vi "Write Boolean Value.vi"(8 "error in (no error)":errorcluster, 10 "Visible?":bool, 11 "Boolean Assertion in":refnum<class "Boolean Assertion.lvclass">) -> (0 "error out":errorcluster, 3 "Boolean Assertion out":refnum<class "Boolean Assertion.lvclass">)   [LabVIEW 2020, in "MacroAssert.lvlib" / "Boolean Assertion.lvclass"]
uses:
  Boolean Assertion.lvclass
  Boolean Assertion.lvclass/Boolean Assertion.ctl
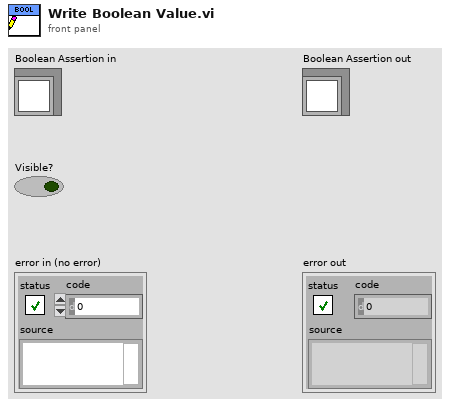
[diagram p1: front panel]
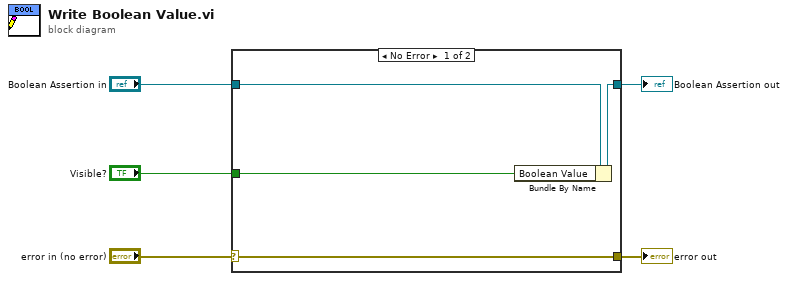
[diagram p0: block diagram]
diagram:
  n1 = case shown="No Error" "error in (no error)" {
    selector: "error in (no error)" -> [w9 w10]
    tunnel: [w9 w10] -> w4
    tunnel: [w7 w11] -> w2
    tunnel: "Boolean Assertion in" -> [w8 w11]
    tunnel: "Visible?" -> [w6 _]
    frame No Error {
      n2 = Bundle By Name(cluster=w8, "Boolean Value"=w6) -> (w7:refnum<class "Boolean Assertion.lvclass">)
    }
    frame Error {
    }
  }
  "error out" <- w4
  "Boolean Assertion out" <- w2
